vi "taskTrial.vi"(4 "mazeDirection":string, 5 "difficulty":dbl, 6 "up or down":string, 7 "Rat ID":string, 8 "error in (no error)":errorcluster, 9 "previousChoices":i32[][](array[numeric]), 10 "Goal \nplatform":i32, 11 "Start \nplatform":i32) -> (0 "error out":errorcluster, 1 "previousChoices updated":i32[][](array[numeric]), 3 "choicesCurrent":i32[][](array[numeric]))   [LabVIEW 2017]
panel:
  out "array w/ subset deleted":i32[](array[numeric])
  out "appended array":i32[](array[numeric])
  out "new\nplatform":i32
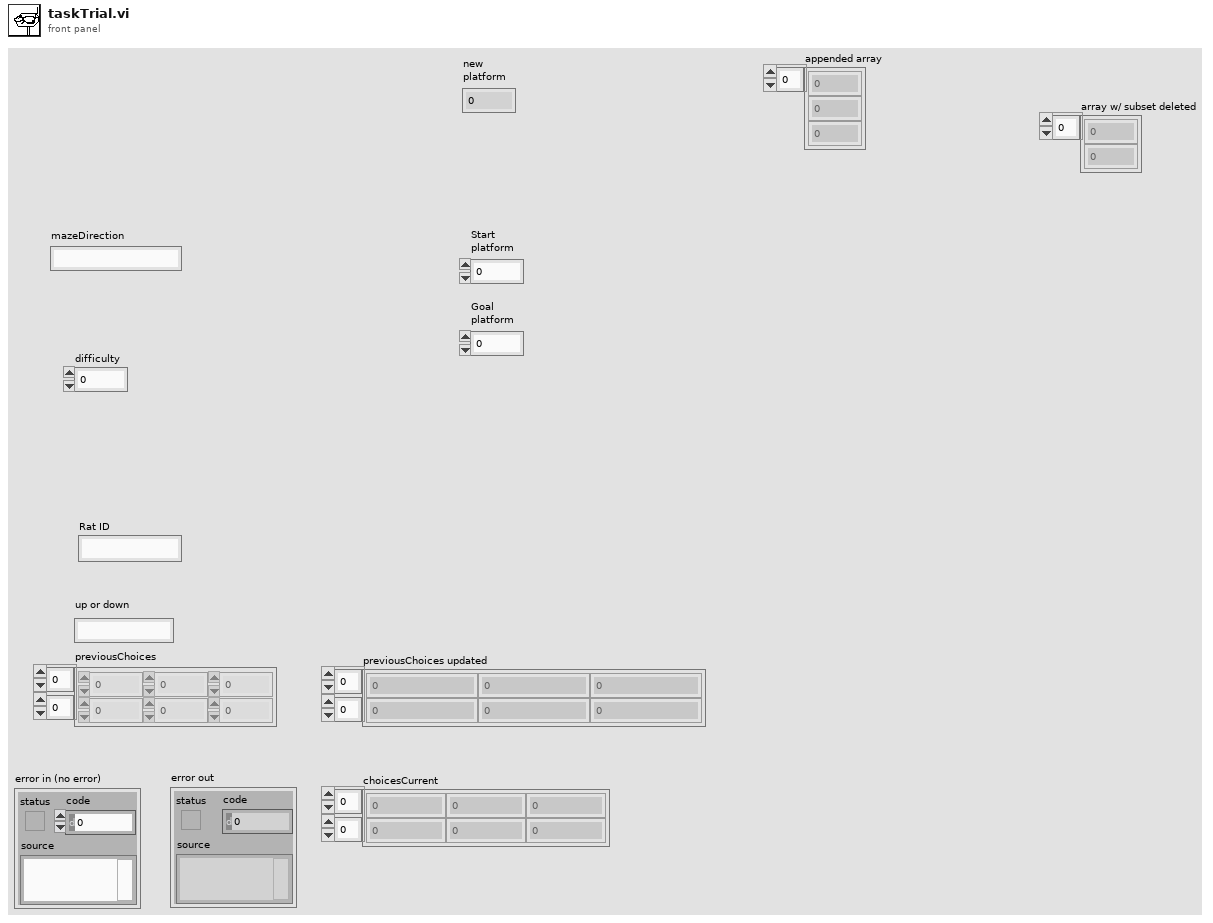
[diagram p1: front panel]
types:
  T1 = enum16{"open", "replace", "create", "open or create", "replace or create", "replace or create with confirmation"}
  T2 = enum16{"big-endian, network order", "native, host order", "little-endian"}
  T3 = cluster{"normal time":dbl, "high res \nrelative time":dbl, "high res \nrelative time":dbl, "Numeric":dbl, "Numeric":dbl, "Numeric":dbl, "vector length":dbl, "vector length":dbl, "vector length":dbl, "vector \nangle":dbl, "vector \nangle":dbl, "vector \nangle":dbl, dbl}
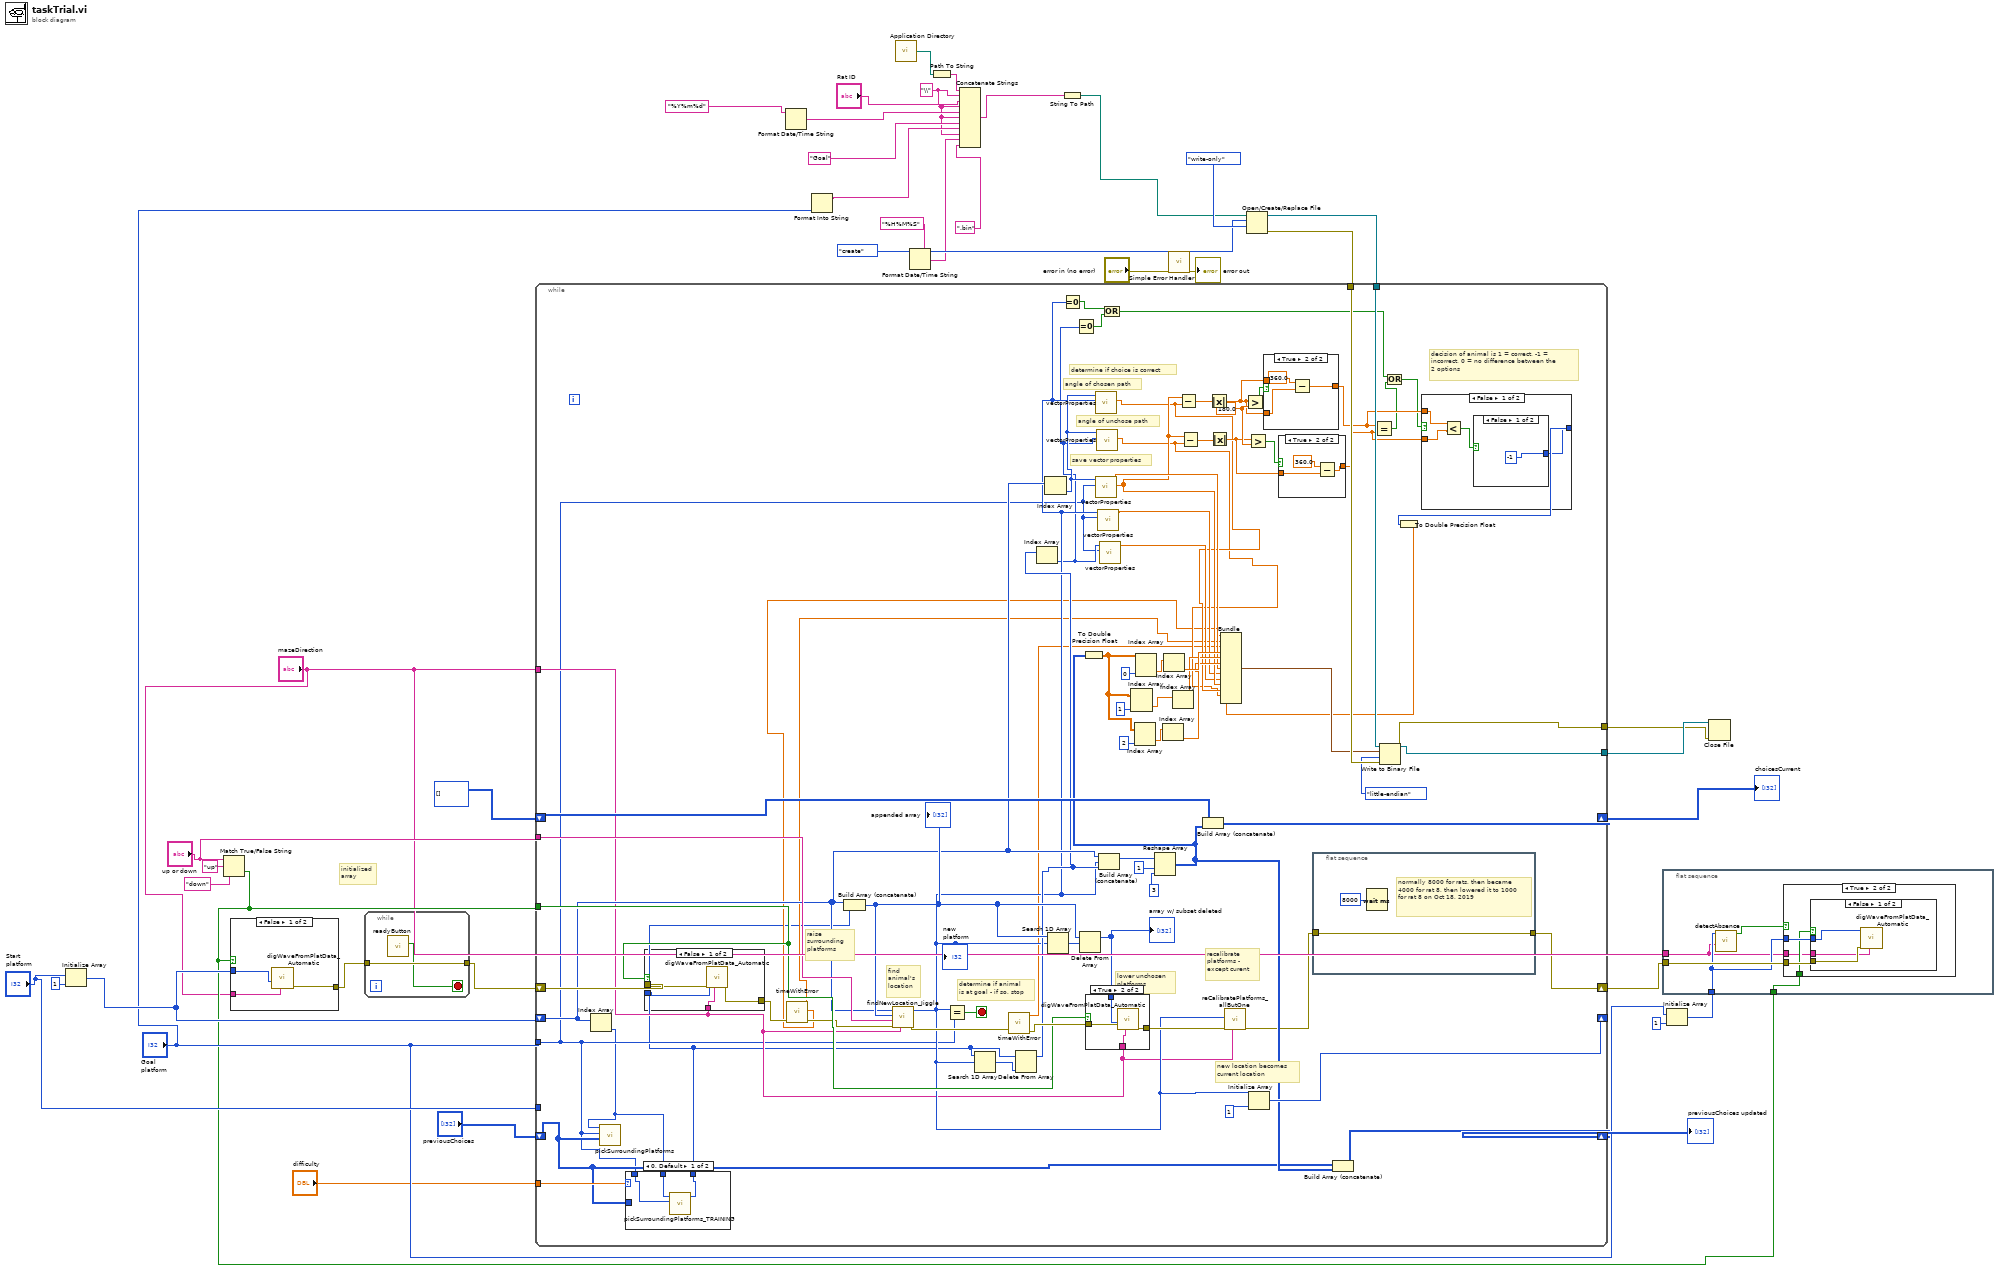
[diagram p0: block diagram]
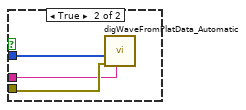
[diagram p3: hidden frame]
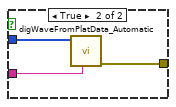
[diagram p4: hidden frame]
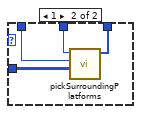
[diagram p5: hidden frame]
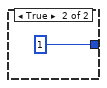
[diagram p6: hidden frame]
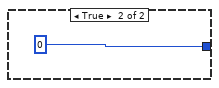
[diagram p7: hidden frame]
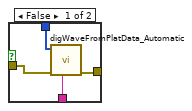
[diagram p10: hidden frame]
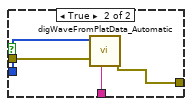
[diagram p11: hidden frame]
diagram:
  w18 = "\\" ("string")
  # "initialized\narray"
  n1 = Initialize Array("Start \nplatform", 1 ("dimension size")) -> (w34:i32[])
  n2 = Match True/False String(2:"down" ("false string"), 3:"up" ("true string"), 4:"up or down") -> (0:w3:bool)  [unwired: 1 out]
  n3 = case shown="False" w3 {
    tunnel: [w43 w46] -> w9
    tunnel: w34 -> [w42 w45]
    tunnel: "mazeDirection" -> [w41 w44]
    frame False {
      n4 = call "digWaveFromPlatData_Automatic.vi"("mazeDirection"=w41, "Platforms\nto lower"=w42) -> ("error out"=w43:errorcluster)  [unwired: 9 in]
    }
    frame True {
      n5 = call "digWaveFromPlatData_Automatic.vi"("mazeDirection"=w44, "Platforms\nto raise"=w45) -> ("error out"=w46:errorcluster)  [unwired: 9 in]
    }
  }
  n6 = while {
    tunnel: w9 -> [w48]
    tunnel: [w48] -> w8
    stop <- w47 stop-if-true
    n7 = call "readyButton.vi"() -> ("Ready? 2"=w47:bool)  [unwired: 9 in]
  }
  n8 = Format Date/Time String(time format string (%c)="%Y%m%d" ("time string")) -> (date/time string=w20:string)  [unwired: 2 in]
  n9 = Format Into String("Goal \nplatform") -> (resulting string=w21:string)  [unwired: 3 in, 1 out]
  n10 = call <vilib>:"Application Directory.vi"() -> ("Application Directory"=w23:path)
  n11 = Format Date/Time String(time format string (%c)="%H%M%S" ("time string")) -> (date/time string=w16:string)  [unwired: 2 in]
  n12 = Path To String(path=w23) -> (string=w26:string)
  n13 = Concatenate Strings(w26, w18, "Rat ID", w18, w20, w18, "Goal" ("string"), w21, w18, w16, ".bin") -> (w14:string)
  n14 = String To Path(string=w14) -> (path=w22:path)
  n15 = call <vilib>:"Simple Error Handler.vi"("error in (no error)"="error in (no error)") -> ("error out"=→"error out":errorcluster)  [unwired: 4 in, 4 out]
  n16 = Open/Create/Replace File(file path (use dialog)=w22, operation (0:open)=T1."create", access (0:read/write)=enum16{"read/write", "read-only", "write-only"}."write-only") -> (refnum out=w30:refnum<file>, error out=w29:errorcluster)  [unwired: 3 in, 1 out]
  n17 = while {
    tunnel: "Goal \nplatform" -> [w51]
    shift-right: [w87] -> w7
    shift-left: w8 -> [w119]
    shift-right: [w110] -> w39
    shift-left: i32[][] [] -> [w118]
    shift-right: [w114] -> w38
    shift-left: "previousChoices" -> [w52]
    shift-right: [w113] -> _
    shift-left: w34 -> [w86]
    tunnel: w30 -> [w109]
    tunnel: w29 -> [w108]
    tunnel: [w106] -> w28
    tunnel: [w105] -> w27
    tunnel: w3 -> [w89]
    tunnel: "up or down" -> [w90]
    tunnel: "Start \nplatform" -> [_]
    tunnel: "mazeDirection" -> [w54]
    tunnel: "difficulty" -> [w53]
    stop <- w122 stop-if-true
    w81 = 180.0 ("y")
    # "decision of animal is 1 = correct, -1 = \nincorrect, 0 = no difference between the \n2 options"
    # "angle of unchose path"
    # "angle of chosen path"
    # "save vector properties"
    # "determine if choice is correct"
    # "determine if animal \nis at goal - if so, stop"
    # "new location becomes\ncurrent location"
    # "recalibrate \nplatforms - \nexcept curent"
    # "lower unchosen\nplatforms"
    # "find \nanimal's \nlocation"
    # "raise \nsurrounding \nplatforms"
    n18 = Index Array(array=w86) -> (element=w50:i32)  [unwired: 1 in]
    n19 = call "pickSurroundingPlatforms.vi"("previousChoices"=w52, "Goal \nplatform"=w51, "Start platform"=w50) -> ()  [unwired: 8 in, 1 out]
    n20 = case shown="0, Default" w53 {
      tunnel: w52 -> [_ w131]
      tunnel: w51 -> [w127 w130]
      tunnel: w50 -> [w125 w129]
      tunnel: [w126 w128] -> w49
      frame 0, Default {
        n21 = call "pickSurroundingPlatforms_TRAINING.vi"("Goal \nplatform"=w127, "Start platform"=w125) -> ("platform choices"=w126:i32[])  [unwired: 9 in]
      }
      frame 1 {
        n22 = call "pickSurroundingPlatforms.vi"("previousChoices"=w131, "Goal \nplatform"=w130, "Start platform"=w129) -> ("platform choices"=w128:i32[])  [unwired: 8 in]
      }
    }
    n23 = case shown="False" w89 {
      tunnel: w119 -> [w159 w164]
      tunnel: [w158 w163] -> w59
      tunnel: w49 -> [w160 w162]
      tunnel: w54 -> [w157 w161]
      frame False {
        n24 = call "digWaveFromPlatData_Automatic.vi"("mazeDirection"=w157, "error in (no error)"=w159, "Platforms\nto lower"=w160) -> ("error out"=w158:errorcluster)  [unwired: 8 in]
      }
      frame True {
        n25 = call "digWaveFromPlatData_Automatic.vi"("mazeDirection"=w161, "error in (no error)"=w164, "Platforms\nto raise"=w162) -> ("error out"=w163:errorcluster)  [unwired: 8 in]
      }
    }
    n26 = call "timeWithError.vi"("error in (no error)"=w59) -> ("high res \nrelative time"=w57:dbl, "normal time"=w56:dbl, "error out"=w58:errorcluster)  [unwired: 7 in]
    n27 = Build Array (concatenate)(w86, w49) -> (w112:i32[])
    "appended array" <- w112
    n28 = call "findNewLocation_Jiggle.vi"("mazeDirection"=w54, "error in (no error)"=w58, "up or down"=w90, "possible \nlocations"=w112, "start \nlocation"=w86) -> ("error out"=w91:errorcluster, "new\nplatform"=w72:i32)  [unwired: 5 in]
    "new\nplatform" <- w72
    n29 = Equal?(x=w72, y=w51) -> (x = y?=w122:bool)
    n30 = Search 1D Array(1D array=w49, element=w72) -> (index of element=w111:i32)  [unwired: 1 in]
    n31 = call "timeWithError.vi"("error in (no error)"=w91) -> ("high res \nrelative time"=w55:dbl, "error out"=w92:errorcluster)  [unwired: 7 in, 1 out]
    n32 = Delete From Array(array=w49, index=w111) -> (array with subset deleted=w85:i32[])  [unwired: 1 in, 1 out]
    n33 = Index Array(array=w85) -> (element=w71:i32)  [unwired: 1 in]
    n34 = Index Array(array=w86) -> (element=w84:i32)  [unwired: 1 in]
    n35 = Search 1D Array(1D array=w112, element=w72) -> (index of element=w124:i32)  [unwired: 1 in]
    n36 = Equal To 0?(x=w72) -> (x = 0?=w69:bool)
    n37 = Equal To 0?(x=w71) -> (x = 0?=w70:bool)
    n38 = Delete From Array(array=w112, index=w124) -> (array with subset deleted=w123:i32[])  [unwired: 1 in, 1 out]
    "array w/ subset deleted" <- w123
    n39 = case shown="True" w89 {
      tunnel: w123 -> [w152 w156]
      tunnel: [w150 w155] -> w120
      tunnel: w92 -> [w151 w154]
      tunnel: w54 -> [w149 w153]
      frame False {
        n40 = call "digWaveFromPlatData_Automatic.vi"("mazeDirection"=w149, "error in (no error)"=w151, "Platforms\nto raise"=w152) -> ("error out"=w150:errorcluster)  [unwired: 8 in]
      }
      frame True {
        n41 = call "digWaveFromPlatData_Automatic.vi"("mazeDirection"=w153, "error in (no error)"=w154, "Platforms\nto lower"=w156) -> ("error out"=w155:errorcluster)  [unwired: 8 in]
      }
    }
    n42 = call "vectorProperties.vi"("Goal \nplatform"=w72, "Start \nplatform"=w84) -> ("vector \nangle"=w61:dbl)  [unwired: 8 in, 1 out]
    n43 = call "vectorProperties.vi"("Goal \nplatform"=w51, "Start \nplatform"=w84) -> ("vector \nangle"=w64:dbl, "vector length"=w65:dbl)  [unwired: 8 in]
    n44 = call "vectorProperties.vi"("Goal \nplatform"=w71, "Start \nplatform"=w84) -> ("vector \nangle"=w60:dbl)  [unwired: 8 in, 1 out]
    n45 = call "vectorProperties.vi"("Goal \nplatform"=w51, "Start \nplatform"=w72) -> ("vector length"=w63:dbl)  [unwired: 8 in, 1 out]
    n46 = Build Array (concatenate)(w86, w72, w85) -> (w115:i32[])
    n47 = call "vectorProperties.vi"("Goal \nplatform"=w51, "Start \nplatform"=w71) -> ("vector length"=w62:dbl)  [unwired: 8 in, 1 out]
    n48 = Or(x=w69, y=w70) -> (x .or. y?=w68:bool)
    n49 = Reshape Array(w115, 1 ("dimension size"), 3 ("dimension size")) -> (w104:i32[][])
    n50 = To Double Precision Float(number=w104) -> (double precision float=w98:dbl[][])
    n51 = Index Array(array=w98, index (col)=1 ("disabled index (col)")) -> (element=w99:dbl[])  [unwired: 1 in]
    n52 = Index Array(array=w98, index (col)=2 ("disabled index (col)")) -> (element=w96:dbl[])  [unwired: 1 in]
    n53 = Index Array(array=w98, index (col)=0 ("disabled index (col)")) -> (element=w102:dbl[])  [unwired: 1 in]
    n54 = Index Array(array=w96) -> (element=w94:dbl)  [unwired: 1 in]
    n55 = Index Array(array=w102) -> (element=w101:dbl)  [unwired: 1 in]
    n56 = Index Array(array=w99) -> (element=w95:dbl)  [unwired: 1 in]
    n57 = Subtract(x=w64, y=w61) -> (x-y=w83:dbl)
    n58 = Subtract(x=w64, y=w60) -> (x-y=w82:dbl)
    n59 = Build Array (concatenate)(w118, w104) -> (w110:i32[][])
    n60 = Absolute Value(x=w83) -> (abs(x)=w79:dbl)
    n61 = Absolute Value(x=w82) -> (abs(x)=w77:dbl)
    n62 = call "reCalibratePlatforms_allButOne.vi"("mazeDirection"=w54, "error in (no error)"=w120, "Current location"=w72) -> ("error out"=w88:errorcluster)  [unwired: 8 in]
    n63 = Greater?(x=w79, y=w81) -> (0:w80:bool)
    n64 = Greater?(x=w77, y=w81) -> (0:w78:bool)
    n65 = Initialize Array(w72, 1 ("dimension size")) -> (w113:i32[])
    n66 = case shown="True" w80 {
      tunnel: w79 -> [_ w145]
      tunnel: [w143 w144] -> w76
      tunnel: w79 -> [w143 _]
      frame False {
      }
      frame True {
        n67 = Subtract(x=360.0, y=w145) -> (x-y=w144:dbl)
      }
    }
    n68 = case shown="True" w78 {
      tunnel: w77 -> [w139 w141]
      tunnel: [w139 w140] -> w75
      frame False {
      }
      frame True {
        n69 = Subtract(x=360.0, y=w141) -> (x-y=w140:dbl)
      }
    }
    n70 = flat-sequence {
      tunnel: w88 -> [w148]
      tunnel: [w148] -> w87
      frame #0 {
        # "normally 8000 for rats, then became 4000 for rat 8, then lowered it to 1000 for rat 8 on Oct 18, 2019"
        n71 = Wait (ms)(milliseconds to wait=u32 8000) -> ()  [unwired: 1 out]
      }
    }
    n72 = Build Array (concatenate)(w52, w104) -> (w114:i32[][])
    n73 = Equal?(x=w76, y=w75) -> (x = y?=w67:bool)
    n74 = Or(x=w68, y=w67) -> (x .or. y?=w66:bool)
    n75 = case shown="False" w66 {
      tunnel: [w132 0] -> w74
      tunnel: w76 -> [w135 _]
      tunnel: w75 -> [w134 _]
      frame False {
        n76 = Less?(x=w135, y=w134) -> (x < y?=w133:bool)
        n77 = case shown="False" w133 {
          tunnel: [-1 1] -> w132
          frame False {
          }
          frame True {
          }
        }
      }
      frame True {
      }
    }
    n78 = To Double Precision Float(number=w74) -> (double precision float=w73:dbl)
    n79 = Bundle("normal time"=w56, "high res \nrelative time"=w57, "high res \nrelative time"=w55, "Numeric"=w101, "Numeric"=w95, "Numeric"=w94, "vector length"=w65, "vector length"=w63, "vector length"=w62, "vector \nangle"=w64, "vector \nangle"=w61, "vector \nangle"=w60, w73) -> (w93:T3)  [unwired: 1 in]
    n80 = Write to Binary File(file (use dialog)=w109, data=w93, error in=w108, 9:T2."little-endian" ("byte order (0:big-endian, network order)")) -> (refnum out=w106:refnum<file>, error out=w105:errorcluster)  [unwired: 2 in, 1 out]
  }
  "choicesCurrent" <- w39
  "previousChoices updated" <- w38
  n81 = flat-sequence {
    tunnel: w7 -> [w169]
    tunnel: w4 -> [w168]
    tunnel: w3 -> [w166]
    tunnel: "mazeDirection" -> [w165]
    frame #0 {
      n82 = call "detectAbsence.vi"("mazeDirection"=w165, "platforms"=w168) -> ("Boolean"=w167:bool)  [unwired: 9 in]
      n83 = case shown="True" w167 {
        tunnel: w169 -> [_ w173]
        tunnel: w168 -> [_ w172]
        tunnel: w166 -> [_ w171]
        tunnel: w165 -> [_ w170]
        frame False {
        }
        frame True {
          n84 = case shown="False" w171 {
            tunnel: w173 -> [w175 w179]
            tunnel: w172 -> [w176 w178]
            tunnel: w170 -> [w174 w177]
            frame False {
              n85 = call "digWaveFromPlatData_Automatic.vi"("mazeDirection"=w174, "error in (no error)"=w175, "Platforms\nto raise"=w176) -> ()  [unwired: 8 in, 1 out]
            }
            frame True {
              n86 = call "digWaveFromPlatData_Automatic.vi"("mazeDirection"=w177, "error in (no error)"=w179, "Platforms\nto lower"=w178) -> ()  [unwired: 8 in, 1 out]
            }
          }
        }
      }
    }
  }
  n87 = Initialize Array("Goal \nplatform", 1 ("dimension size")) -> (w4:i32[])
  n88 = Close File(refnum=w28, error in=w27) -> ()  [unwired: 2 out]
